vi "Set-Image-height.vi"(8 "error in (no error)":errorcluster, 10 "Image height in":i32, 11 "Camera in":refnum<class "Camera.lvclass">) -> (0 "error out":errorcluster, 1 "Image height offset":i32, 2 "Image height":i32, 3 "Camera out":refnum<class "Camera.lvclass">)   [LabVIEW 2013, in "CameraVision.lvlib" / "Camera.lvclass"]
uses:
  Camera.lvclass
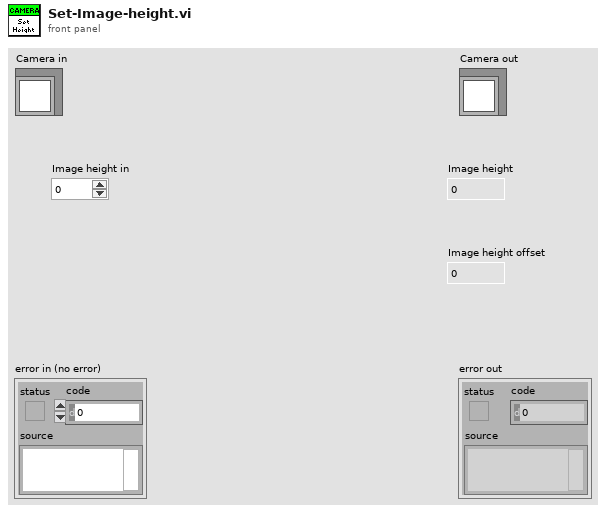
[diagram p1: front panel]
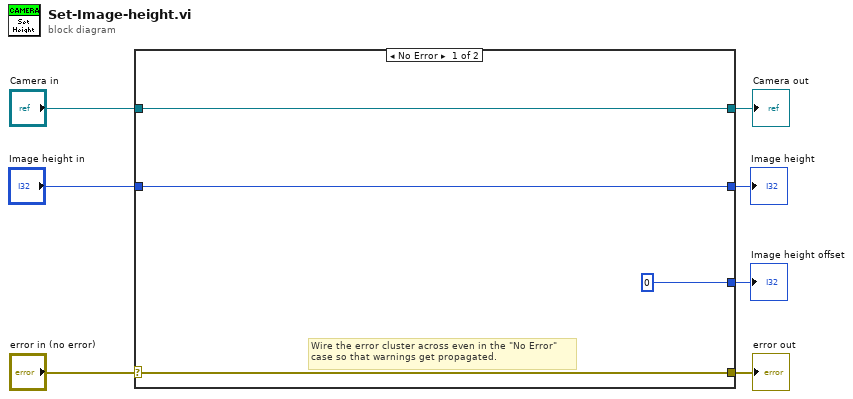
[diagram p0: block diagram]
diagram:
  n1 = case shown="No Error" "error in (no error)" {
    selector: "error in (no error)" -> [w10 w14]
    tunnel: [w10 w14] -> w6
    tunnel: [w11 w13] -> w4
    tunnel: "Camera in" -> [w11 w13]
    tunnel: [w9 w12] -> w2
    tunnel: "Image height in" -> [w9 w12]
    tunnel: [0 _] -> w1
    frame No Error {
      # "Wire the error cluster across even in the \"No Error\"\ncase so that warnings get propagated."
    }
    frame Error {
    }
  }
  "error out" <- w6
  "Camera out" <- w4
  "Image height" <- w2
  "Image height offset" <- w1
